vi "sid_output_binaryMem.vi"(6 "inputValid":bool, 7 "startId":bool, 9 "sysIdParams":T1={"sysIdOutputRate"=100, "sysIdWaveSize"=4092, "sysIdRepetitions"=50, "high"=0.0, "low"=0.0} {"sysIdOutputRate" min=10}, 11 "feedbackHeight":fxp<+/-,28,1>) -> (0 "sysIdRunning":bool, 1 "recordPoint":bool, 2 "sysIdRep":u16, 3 "sid.o.height":fxp<+/-,28,1>, 4 "outputValid":bool, 5 "sysIdWaveIndex":u16)   [LabVIEW 2016]
uses:
  <vilib>/rvi/Memory/Memory_Emulation/nirvimemoryFastEmulation.vi
  <vilib>/rvi/Memory/Memory_Emulation/nirvimemoryEmulation.vi
  <vilib>/rvi/Emulation/niFpgaEmulationIsFPGAContextNoSignature.vi
  <vilib>/rvi/DataTransferAndStorage/Container/Common/niFpgaContainerGetUniqueNameForEmu.vi
  <vilib>/rvi/Emulation/niFpgaProcessEmulError.vi
  <vilib>/rvi/Emulation/niFpgaSctlEmulationGetInTimedLoop.vi
  <vilib>/rvi/errors/nirviReportUnexpectedCaseInternalError (U32).vi
  <vilib>/rvi/DataTransferAndStorage/Container/XNode/niFpgaContainer.xnode
  <vilib>/rvi/FXPMathLib/FxpAdd/XNode/nifxpmath_Add.xnode
  <instrlib>/_niInstr/Basic Elements/v1/FPGA/niInstr Basic Elements v1 FPGA.lvlib
  <vilib>/rvi/FXPMathLib/sim/FxpSim.dll
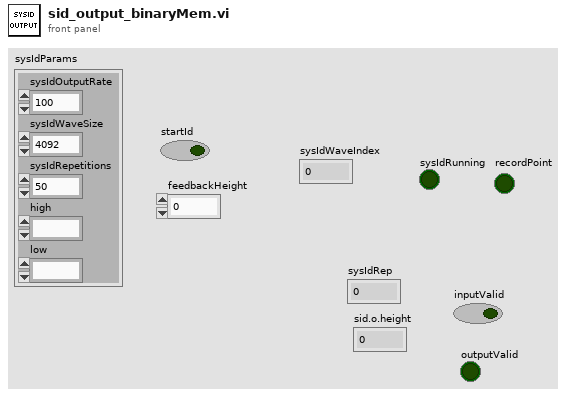
[diagram p1: front panel]
types:
  T1 = cluster{"sysIdOutputRate":u16, "sysIdWaveSize":u16, "sysIdRepetitions":u16, "high":fxp<+/-,17,1>, "low":fxp<+/-,17,1>}
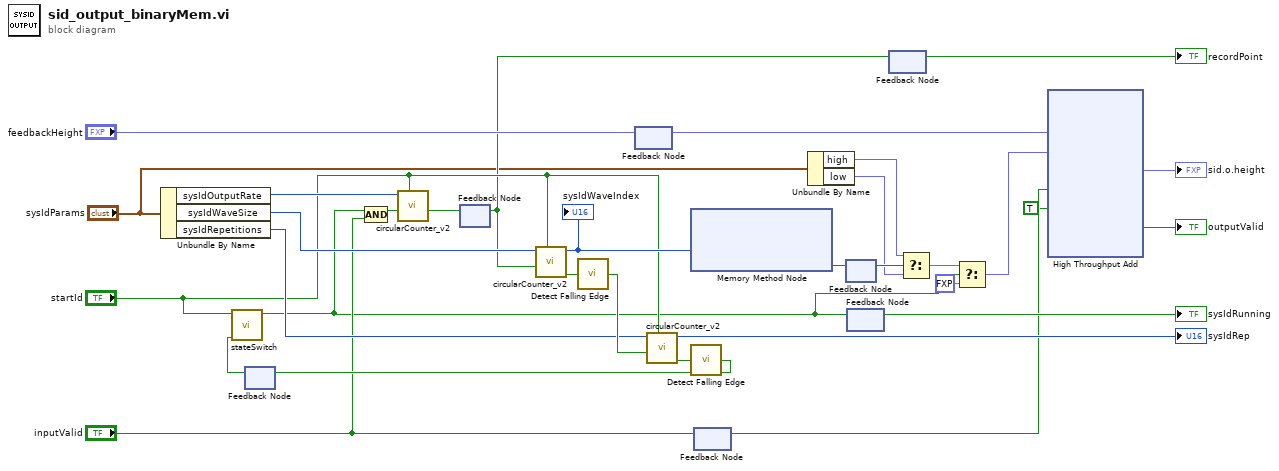
[diagram p0: block diagram]
diagram:
  n1 = Unbundle By Name("sysIdParams") -> ("sysIdOutputRate"=w25:u16, "sysIdWaveSize"=w24:u16, "sysIdRepetitions"=w23:u16)
  n2 = feedback #1() -> (w27:bool)  [unwired: 1 in]
  n3 = call "stateSwitch.vi"("disable"=w27, "enable"="startId") -> ("state"=w5:bool)  [unwired: 9 in]
  n4 = Compound Arithmetic op=AND(w5, "inputValid") -> (w15:bool)
  n5 = call "circularCounter_v2.vi"("reset"="startId", "doStep"=w15, "maxCount"=w25) -> ("maxPulse"=w16:bool)  [unwired: 5 in, 3 out]
  n6 = feedback-in #2(w16) -> ()
  n7 = feedback #2() -> (w14:bool)  [unwired: 1 in]
  n8 = call "circularCounter_v2.vi"("reset"="startId", "doStep"=w14, "maxCount"=w24) -> ("maxReached"=w31:bool, "index"=w32:u16)  [unwired: 5 in, 2 out]
  "sysIdWaveIndex" <- w32
  n9 = call <instrlib>:"Detect Falling Edge.vi"("signal"=w31) -> ("edge detected"=w30:bool)  [unwired: 14 in]
  n10 = feedback-in #3("feedbackHeight") -> ()
  n11 = feedback #3() -> (w7:fxp<+/-,28,1>)  [unwired: 1 in]
  n12 = call "circularCounter_v2.vi"("reset"="startId", "doStep"=w30, "maxCount"=w23) -> ("maxReached"=w29:bool, "index"=→"sysIdRep":u16)  [unwired: 5 in, 2 out]
  n13 = xnode ("Memory Method Node")("Address"=w32) -> ("Data"=w26:bool)  [unwired: 1 in, 1 out]
  n14 = call <instrlib>:"Detect Falling Edge.vi"("signal"=w29) -> ("edge detected"=w28:bool)  [unwired: 14 in]
  n15 = feedback-in #1(w28) -> ()
  n16 = feedback #4() -> (w12:bool)  [unwired: 1 in]
  n17 = feedback-in #4("inputValid") -> ()
  n18 = Unbundle By Name("sysIdParams") -> ("high"=w2:fxp<+/-,17,1>, "low"=w1:fxp<+/-,17,1>)
  n19 = feedback #5() -> (w10:bool)  [unwired: 1 in]
  n20 = feedback-in #5(w26) -> ()
  n21 = feedback #6() -> (→"sysIdRunning":bool)  [unwired: 1 in]
  n22 = feedback-in #6(w5) -> ()
  n23 = feedback-in #7(w14) -> ()
  n24 = feedback #7() -> (→"recordPoint":bool)  [unwired: 1 in]
  n25 = Select(t=w2, s=w10, f=w1) -> (s? t:f=w9:fxp<+/-,17,1>)
  n26 = Select(t=w9, s=w5, f=fxp<+/-,16,1> 0.0) -> (s? t:f=w6:fxp<+/-,17,1>)
  n27 = xnode ("High Throughput Add")("x"=w7, "y"=w6, "input valid"=w12, "ready for output (T)"=TRUE) -> ("x+y"=→"sid.o.height":fxp<+/-,28,1>, "output valid"=→"outputValid":bool)  [unwired: 1 out]
